vi "RichToFlatcif_manager_PluginInfoResponse.vi"(5 "OutputClusterType":T1, 11 "InputCluster":T14) -> (3 "OutputCluster":T1)   [LabVIEW 2021, in "CIF_PluginLoader_client.lvlib"]
uses:
  cif_manager_PluginInfoResponse.ctl
  cif_manager_PluginInfo.ctl
  cif_common_ShortVersion.ctl
  cif_plugincore_StatusData.ctl
  cif_plugincore_StatusData_PluginState.ctl
  cif_plugincore_TimingStatistics.ctl
  cif_common_TimingStats.ctl
  cif_plugincore_FifoStatistics.ctl
  cif_plugincore_Error.ctl
  cif_plugincore_MonitorDoubles.ctl
  cif_plugincore_MonitorU64.ctl
  cif_plugincore_MonitorI64.ctl
  cif_common_Status.ctl
  cif_manager_PluginInfoResponse_Flat.ctl
  cif_manager_PluginInfo_Flat.ctl
  cif_common_ShortVersion_Flat.ctl
  cif_plugincore_StatusData_Flat.ctl
  cif_plugincore_TimingStatistics_Flat.ctl
  cif_common_TimingStats_Flat.ctl
  cif_plugincore_FifoStatistics_Flat.ctl
  cif_plugincore_Error_Flat.ctl
  cif_plugincore_MonitorDoubles_Flat.ctl
  cif_plugincore_MonitorU64_Flat.ctl
  cif_plugincore_MonitorI64_Flat.ctl
  cif_common_Status_Flat.ctl
  CIF_PluginLoader_client.lvlib
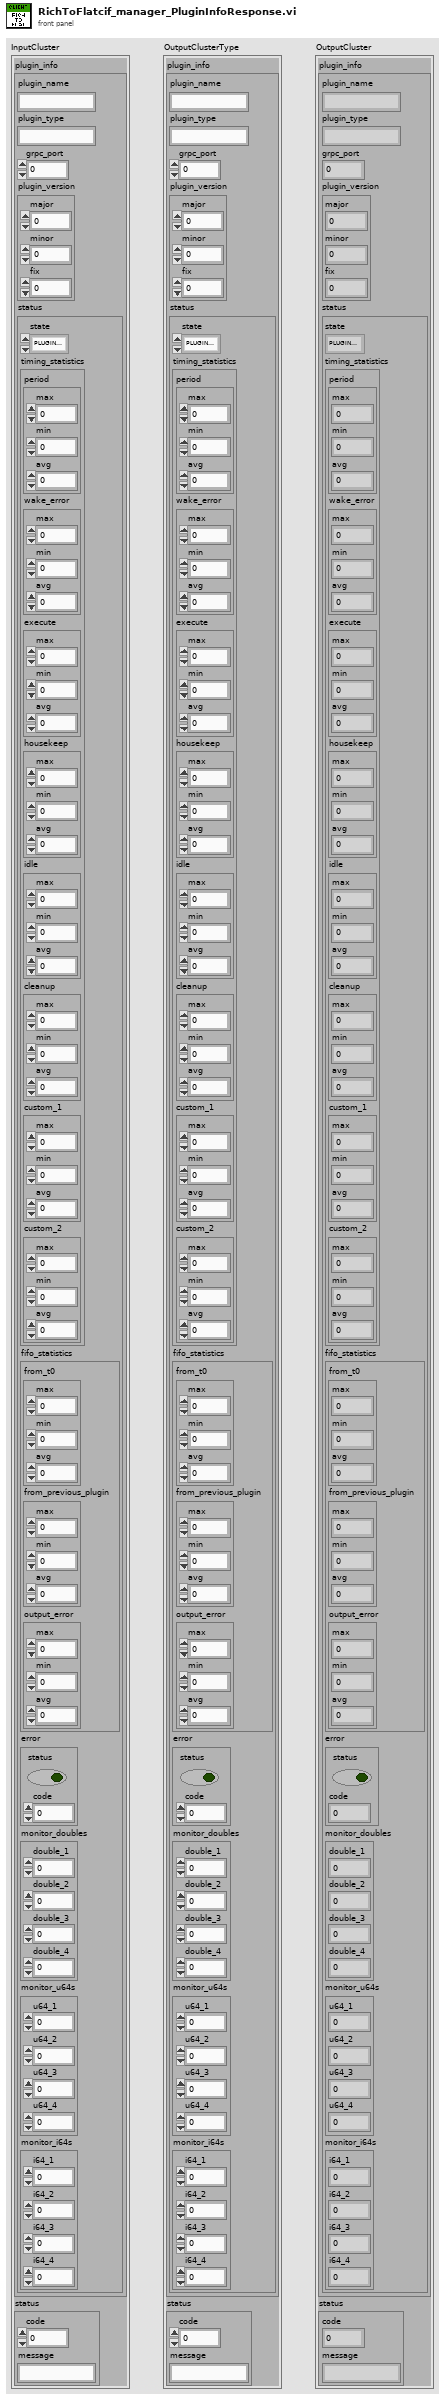
[diagram p1: front panel]
types:
  T1 = typedef "CIF_PluginLoader_client.lvlib/cif_manager_PluginInfoResponse_Flat.ctl" = cluster{"plugin_info":T2, "status":T13}
  T2 = typedef "CIF_PluginLoader_client.lvlib/cif_manager_PluginInfo_Flat.ctl" = cluster{"plugin_name":string, "plugin_type":string, "grpc_port":i32, "plugin_version":T3, "status":T4}
  T3 = typedef "CIF_PluginLoader_client.lvlib/cif_common_ShortVersion_Flat.ctl" = cluster{"major":u32, "minor":u32, "fix":u32}
  T4 = typedef "CIF_PluginLoader_client.lvlib/cif_plugincore_StatusData_Flat.ctl" = cluster{"state":T5, "timing_statistics":T6, "fifo_statistics":T8, "error":T9, "monitor_doubles":T10, "monitor_u64s":T11, "monitor_i64s":T12}
  T5 = typedef "CIF_PluginLoader_client.lvlib/cif_plugincore_StatusData_PluginState.ctl" = enum32{"PLUGINSTATE_UNKNOWN", "PLUGINSTATE_CREATING", "PLUGINSTATE_LISTENING", "PLUGINSTATE_RUNNING", "PLUGINSTATE_CLEANINGUP", "PLUGINSTATE_DESTROYING"}
  T6 = typedef "CIF_PluginLoader_client.lvlib/cif_plugincore_TimingStatistics_Flat.ctl" = cluster{"period":T7, "wake_error":T7, "execute":T7, "housekeep":T7, "idle":T7, "cleanup":T7, "custom_1":T7, "custom_2":T7}
  T7 = typedef "CIF_PluginLoader_client.lvlib/cif_common_TimingStats_Flat.ctl" = cluster{"max":i64, "min":i64, "avg":dbl}
  T8 = typedef "CIF_PluginLoader_client.lvlib/cif_plugincore_FifoStatistics_Flat.ctl" = cluster{"from_t0":T7, "from_previous_plugin":T7, "output_error":T7}
  T9 = typedef "CIF_PluginLoader_client.lvlib/cif_plugincore_Error_Flat.ctl" = cluster{"status":bool, "code":i32}
  T10 = typedef "CIF_PluginLoader_client.lvlib/cif_plugincore_MonitorDoubles_Flat.ctl" = cluster{"double_1":dbl, "double_2":dbl, "double_3":dbl, "double_4":dbl}
  T11 = typedef "CIF_PluginLoader_client.lvlib/cif_plugincore_MonitorU64_Flat.ctl" = cluster{"u64_1":u64, "u64_2":u64, "u64_3":u64, "u64_4":u64}
  T12 = typedef "CIF_PluginLoader_client.lvlib/cif_plugincore_MonitorI64_Flat.ctl" = cluster{"i64_1":i64, "i64_2":i64, "i64_3":i64, "i64_4":i64}
  T13 = typedef "CIF_PluginLoader_client.lvlib/cif_common_Status_Flat.ctl" = cluster{"code":i32, "message":string}
  T14 = typedef "CIF_PluginLoader_client.lvlib/cif_manager_PluginInfoResponse.ctl" = cluster{"plugin_info":T15, "status":T25}
  T15 = typedef "CIF_PluginLoader_client.lvlib/cif_manager_PluginInfo.ctl" = cluster{"plugin_name":string, "plugin_type":string, "grpc_port":i32, "plugin_version":T16, "status":T17}
  T16 = typedef "CIF_PluginLoader_client.lvlib/cif_common_ShortVersion.ctl" = cluster{"major":u32, "minor":u32, "fix":u32}
  T17 = typedef "CIF_PluginLoader_client.lvlib/cif_plugincore_StatusData.ctl" = cluster{"state":T5, "timing_statistics":T18, "fifo_statistics":T20, "error":T21, "monitor_doubles":T22, "monitor_u64s":T23, "monitor_i64s":T24}
  T18 = typedef "CIF_PluginLoader_client.lvlib/cif_plugincore_TimingStatistics.ctl" = cluster{"period":T19, "wake_error":T19, "execute":T19, "housekeep":T19, "idle":T19, "cleanup":T19, "custom_1":T19, "custom_2":T19}
  T19 = typedef "CIF_PluginLoader_client.lvlib/cif_common_TimingStats.ctl" = cluster{"max":i64, "min":i64, "avg":dbl}
  T20 = typedef "CIF_PluginLoader_client.lvlib/cif_plugincore_FifoStatistics.ctl" = cluster{"from_t0":T19, "from_previous_plugin":T19, "output_error":T19}
  T21 = typedef "CIF_PluginLoader_client.lvlib/cif_plugincore_Error.ctl" = cluster{"status":bool, "code":i32}
  T22 = typedef "CIF_PluginLoader_client.lvlib/cif_plugincore_MonitorDoubles.ctl" = cluster{"double_1":dbl, "double_2":dbl, "double_3":dbl, "double_4":dbl}
  T23 = typedef "CIF_PluginLoader_client.lvlib/cif_plugincore_MonitorU64.ctl" = cluster{"u64_1":u64, "u64_2":u64, "u64_3":u64, "u64_4":u64}
  T24 = typedef "CIF_PluginLoader_client.lvlib/cif_plugincore_MonitorI64.ctl" = cluster{"i64_1":i64, "i64_2":i64, "i64_3":i64, "i64_4":i64}
  T25 = typedef "CIF_PluginLoader_client.lvlib/cif_common_Status.ctl" = cluster{"code":i32, "message":string}
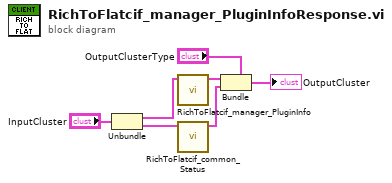
[diagram p0: block diagram]
diagram:
  n1 = Unbundle "Unbundle"("InputCluster") -> ("plugin_info"=w4:T15, "status"=w2:T25)
  n2 = call "RichToFlatcif_manager_PluginInfo.vi"("InputCluster"=w4) -> ("OutputCluster"=w3:T2)  [unwired: 10 in]
  n3 = call "RichToFlatcif_common_Status.vi"("InputCluster"=w2) -> ("OutputCluster"=w1:T13)  [unwired: 10 in]
  n4 = Bundle "Bundle"(cluster="OutputClusterType", "plugin_info"=w3, "status"=w1) -> (→"OutputCluster":T1)
